vi "get Rname.vi"(8 "error in (no error)":errorcluster caption="Fehler (Eingang, kein Fehler)", 11 "Report (Eingang)":refnum<class "Report.lvclass">) -> (0 "error out":errorcluster caption="Fehler (Ausgang)", 2 "Rname":string, 3 "Report (Ausgang)":refnum<class "Report.lvclass">)   [LabVIEW 2013, in "DatenKlassen.lvlib" / "Report.lvclass"]
uses:
  Report.lvclass
  Report.lvclass/Report.ctl
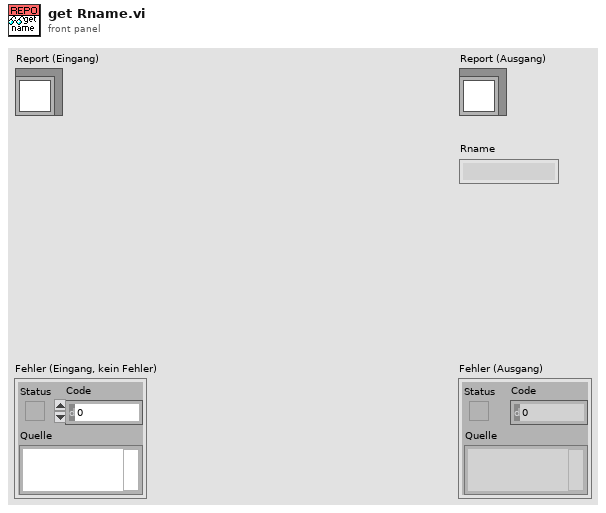
[diagram p1: front panel]
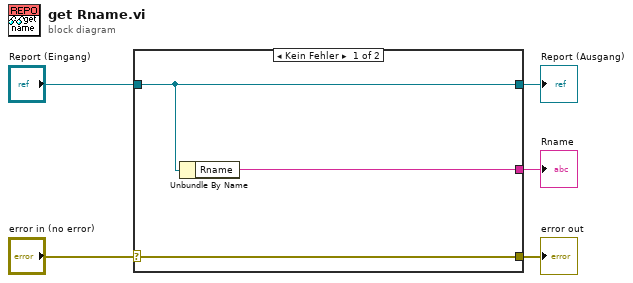
[diagram p0: block diagram]
diagram:
  n1 = case shown="Kein Fehler" "error in (no error)" {
    selector: "error in (no error)" -> [w8 w9]
    tunnel: [w8 w9] -> w4
    tunnel: [w7 w10] -> w2
    tunnel: "Report (Eingang)" -> [w7 w10]
    tunnel: [w6 _] -> w1
    frame No Error {
      n2 = Unbundle By Name(w7) -> ("Rname"=w6:string)
    }
    frame Error {
    }
  }
  "error out" <- w4
  "Report (Ausgang)" <- w2
  "Rname" <- w1
